vi "Configure Bandwidth Limit Test.vi"(0 "VISA resource name":refnum<visa-resource-name>, 1 "Enable Bandwidth Limit Test (F: Disable)":bool, 2 "Bandwidth Threshold Value (3)":dbl=3.0, 5 "Channel (1)":i32=1, 7 "Enable Marker Display (T: Enable)":bool=TRUE, 9 "Enable Bandwidth Display (T: Enable)":bool=TRUE, 11 "error in (no error)":errorcluster, 12 "Lower Limit Value (10000 Hz)":dbl=10000.0, 13 "Upper Limit Value (3E+5 Hz)":dbl=300000.0) -> (4 "VISA resource name out":refnum<visa-resource-name>, 15 "error out":errorcluster)   [LabVIEW 2018, in "Agilent ENA Series.lvlib"]
doc: "Configures the bandwidth limit test.\n\nNote:\nThe control Enable Marker Display does not support model E5080A."
uses:
  Agilent ENA Series.lvlib
panel:
  # "Note:\nThe control Enable Marker Display does not support model E5080A."
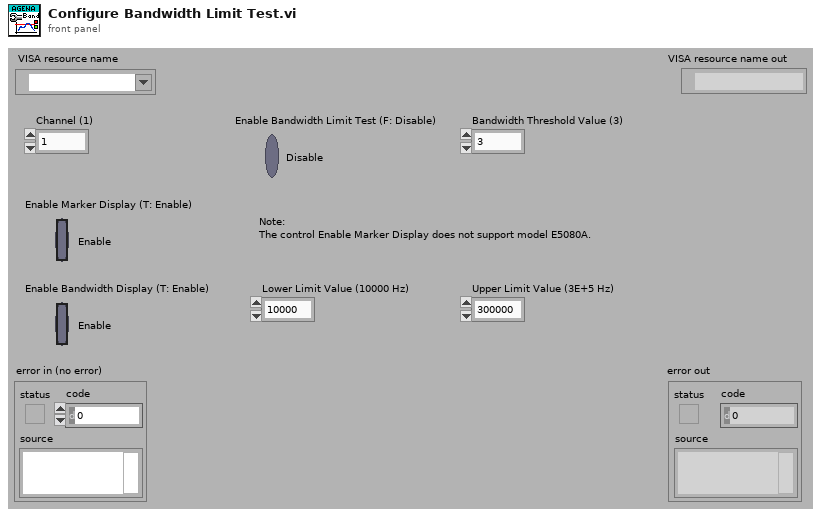
[diagram p1: front panel]
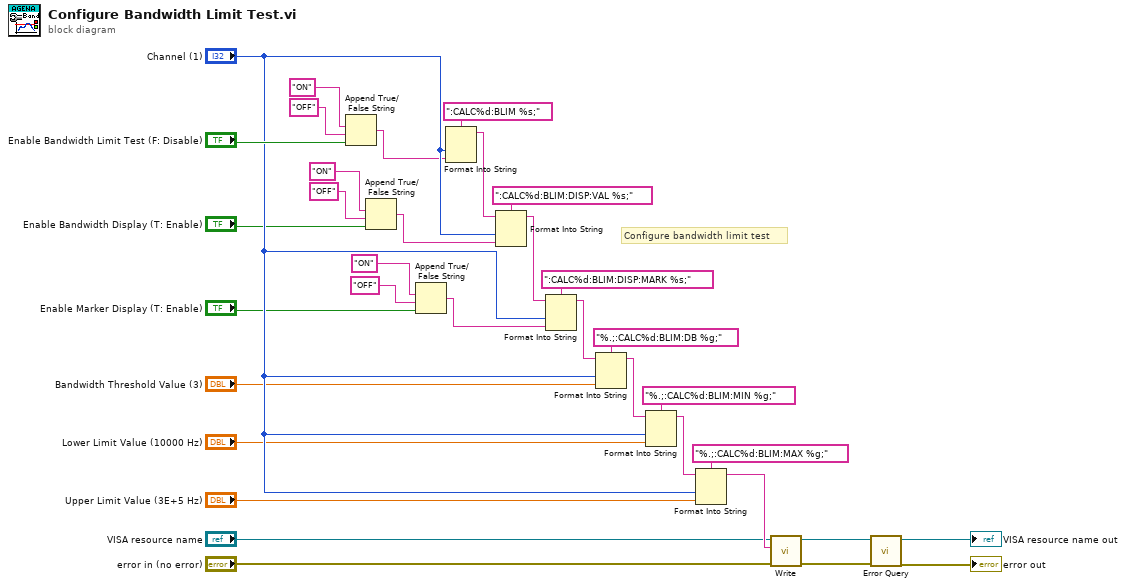
[diagram p0: block diagram]
diagram:
  # "Configure bandwidth limit test"
  n1 = Append True/False String(1:"Enable Bandwidth Limit Test (F: Disable)", 2:"OFF", 3:"ON") -> (0:w29:string)  [unwired: 1 out]
  n2 = Append True/False String(1:"Enable Bandwidth Display (T: Enable)", 2:"OFF", 3:"ON") -> (0:w23:string)  [unwired: 1 out]
  n3 = Append True/False String(1:"Enable Marker Display (T: Enable)", 2:"OFF", 3:"ON") -> (0:w17:string)  [unwired: 1 out]
  n4 = Format Into String(format string=":CALC%d:BLIM %s;", "Channel (1)", w29) -> (resulting string=w25:string)  [unwired: 2 in, 1 out]
  n5 = Format Into String(format string=":CALC%d:BLIM:DISP:VAL %s;", initial string=w25, "Channel (1)", w23) -> (resulting string=w19:string)  [unwired: 1 in, 1 out]
  n6 = Format Into String(format string=":CALC%d:BLIM:DISP:MARK %s;", initial string=w19, "Channel (1)", w17) -> (resulting string=w16:string)  [unwired: 1 in, 1 out]
  n7 = Format Into String(format string="%.;:CALC%d:BLIM:DB %g;", initial string=w16, "Channel (1)", "Bandwidth Threshold Value (3)") -> (resulting string=w13:string)  [unwired: 1 in, 1 out]
  n8 = Format Into String(format string="%.;:CALC%d:BLIM:MIN %g;", initial string=w13, "Channel (1)", "Lower Limit Value (10000 Hz)") -> (resulting string=w10:string)  [unwired: 1 in, 1 out]
  n9 = Format Into String(format string="%.;:CALC%d:BLIM:MAX %g;", initial string=w10, "Channel (1)", "Upper Limit Value (3E+5 Hz)") -> (resulting string=w7:string)  [unwired: 1 in, 1 out]
  n10 = call "Write.vi"("error in (no error)"="error in (no error)", "String ()"=w7, "VISA resource name"="VISA resource name") -> ("error out"=w3:errorcluster, "VISA resource name out"=w4:refnum<visa-resource-name>)  [unwired: 6 in, 1 out]
  n11 = call "Error Query.vi"("error in (no error)"=w3, "VISA resource name"=w4) -> ("error out"=→"error out":errorcluster, "VISA resource name out"=→"VISA resource name out":refnum<visa-resource-name>)  [unwired: 8 out]
